vi "parse_assembly_state_roslv.vi"(0 "Msg in":string, 2 "error in":errorcluster) -> (3 "msg out":string, 4 "Assembly State":T1, 6 "error out":errorcluster)   [LabVIEW 2014]
uses:
  std_msgs/subs/parse_bool_scalar_roslv.vi
  std_msgs/subs/parse_u8_scalar_roslv.vi
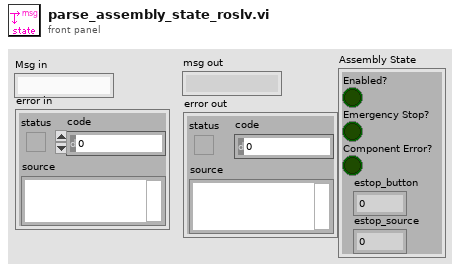
[diagram p1: front panel]
types:
  T1 = cluster{"Enabled?":bool, "Emergency Stop?":bool, "Component Error?":bool, "estop_button":u8, "estop_source":u8}
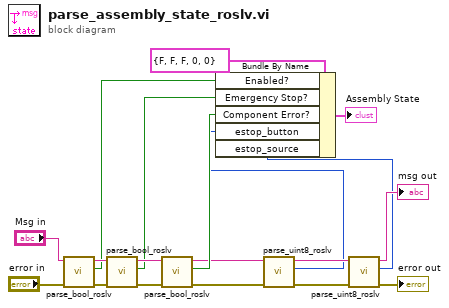
[diagram p0: block diagram]
diagram:
  n1 = call-poly "parse_bool_roslv.vi"("error in"="error in", "msg in"="Msg in") -> ("error out"=w16:errorcluster, "bool"=w14:bool, "msg out"=w19:string)  [unwired: 3 in]
  n2 = call-poly "parse_bool_roslv.vi"("error in"=w16, "msg in"=w19) -> ("error out"=w17:errorcluster, "bool"=w13:bool, "msg out"=w18:string)  [unwired: 3 in]
  n3 = call-poly "parse_bool_roslv.vi"("error in"=w17, "msg in"=w18) -> ("error out"=w8:errorcluster, "bool"=w12:bool, "msg out"=w9:string)  [unwired: 3 in]
  n4 = call-poly "parse_uint8_roslv.vi"("error in"=w8, "msg in"=w9) -> ("error out"=w6:errorcluster, "number"=w3:u8, "msg out"=w7:string)  [unwired: 3 in]
  n5 = call-poly "parse_uint8_roslv.vi"("error in"=w6, "msg in"=w7) -> ("error out"=→"error out":errorcluster, "number"=w2:u8, "msg out"=→"msg out":string)  [unwired: 3 in]
  n6 = Bundle By Name(cluster=T1 {"Enabled?"=FALSE, "Emergency Stop?"=FALSE, "Component Error?"=FALSE, "estop_button"=0, "estop_source"=0} ("input cluster"), "Enabled?"=w14, "Emergency Stop?"=w13, "Component Error?"=w12, "estop_button"=w3, "estop_source"=w2) -> (→"Assembly State":T1)
